vi "PQ Test Get Datatype.vi"(8 "error in (no error)":errorcluster, 10 "Connection String":string="user = llab_reader") -> (0 "error out":errorcluster)   [LabVIEW 2019]
uses:
  <vilib>/addons/_JKI Toolkits/Caraya/classes/Assert/Assert Not Error.vi
  src/LV-Data.PG/LV-Data.PGSQL.lvclass
  <vilib>/addons/_JKI Toolkits/Caraya/classes/Assert/Assert.lvclass
  <vilib>/addons/_JKI Toolkits/Caraya/classes/Test/Test.lvclass
panel:
  out "Datatype":string
  in  "Column Name":string="time"
  in  "Table Path":string="timestamp_demo"
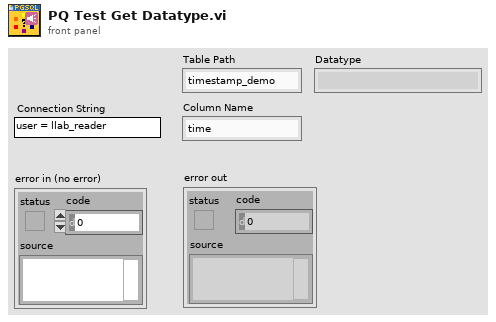
[diagram p1: front panel]
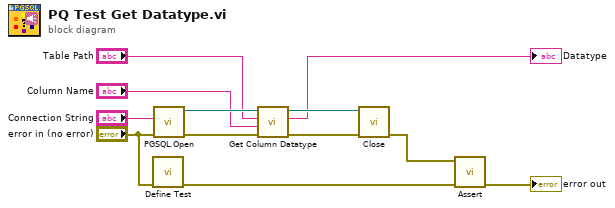
[diagram p0: block diagram]
diagram:
  n1 = call <vilib>:"Define Test.vi"("error in (no error)"="error in (no error)") -> ("error out"=w8:errorcluster)  [unwired: 9 in, 1 out]
  n2 = call "PGSQL.Open.vi"("error in (no error)"="error in (no error)", "Connection String"="Connection String") -> ("error out"=w7:errorcluster, "Data.PG out"=w6:refnum<class "LV-Data.PGSQL.lvclass">)  [unwired: 8 in]
  n3 = call "Get Column Datatype.vi"("error in (no error)"=w7, "Column Name"="Column Name", "Table Path"="Table Path", "LV-Data.PGSQL in"=w6) -> ("error out"=w4:errorcluster, "Datatype"=→"Datatype":string, "LV-Data.PGSQL out"=w5:refnum<class "LV-Data.PGSQL.lvclass">)  [unwired: 5 in]
  n4 = call-dynamic "Close.vi"("error in (no error)"=w4, "Data.PG in"=w5) -> ("error out"=w11:errorcluster)  [unwired: 8 in, 1 out]
  n5 = call-poly <vilib>:"Assert.vi"("error in (no error)"=w8, "Not Error?"=w11) -> ("error out"=→"error out":errorcluster)  [unwired: 8 in, 1 out]
